vi "Generate Executed Tests Fraction String.vi"(8 "error in (no error)":errorcluster, 11 "Coverage Analyzer Result View in":refnum<class "Coverage Analyzer Result View.lvclass">) -> (0 "error out":errorcluster, 2 "Fraction of VIs Executed":string, 3 "Coverage Analyzer Result View out":refnum<class "Coverage Analyzer Result View.lvclass">)   [LabVIEW 2020, in "Coverage Analyzer Result View.lvclass"]
uses:
  Coverage Analyzer Result View.lvclass
  Coverage Analyzer Result View.lvclass/Coverage Analyzer Result View.ctl
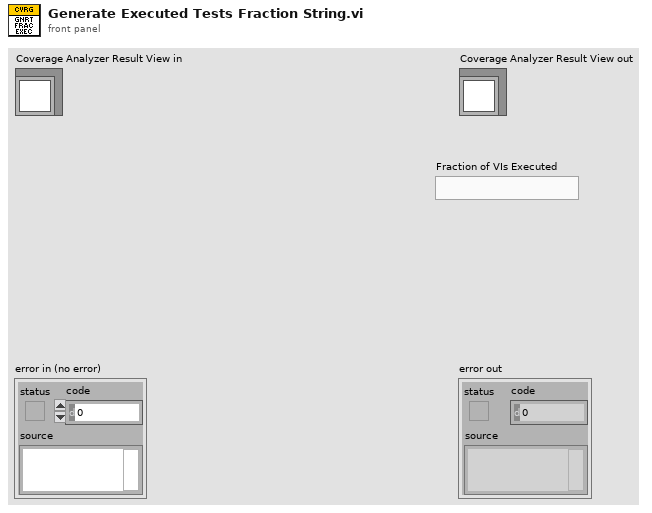
[diagram p1: front panel]
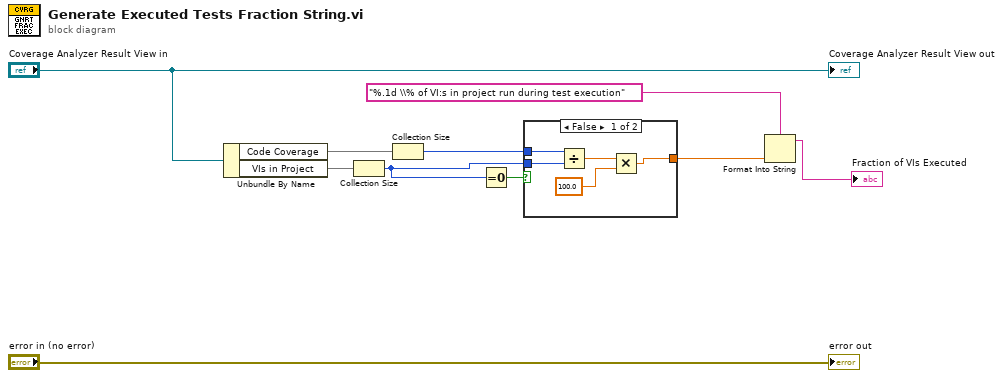
[diagram p0: block diagram]
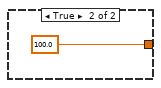
[diagram p2: hidden frame]
diagram:
  n1 = Unbundle By Name("Coverage Analyzer Result View in") -> ("Code Coverage"=w7:map{path, dbl}, "VIs in Project"=w8:set{path})
  n2 = Collection Size(1:w8) -> (0:w3:i32)
  n3 = Collection Size(1:w7) -> (0:w2:i32)
  n4 = Equal To 0?(x=w3) -> (x = 0?=w4:bool)
  n5 = case shown="False" w4 {
    tunnel: w2 -> [w15 _]
    tunnel: [w12 100.0] -> w1
    tunnel: w3 -> [w13 _]
    frame False {
      n6 = Divide(x=w15, y=w13) -> (x/y=w14:dbl)
      n7 = Multiply(x=w14, y=100.0) -> (x*y=w12:dbl)
    }
    frame True {
    }
  }
  n8 = Format Into String(format string="%.1d \\% of VI:s in project run during test execution", w1) -> (resulting string=→"Fraction of VIs Executed":string)  [unwired: 2 in, 1 out]
  "error out" <- "error in (no error)"
  "Coverage Analyzer Result View out" <- "Coverage Analyzer Result View in"
